vi "BINARY_DECIMAL.vi"() -> ()   [LabVIEW 2020]
panel:
  out "DECIMAL VALUE":i16
  in  "B0":bool
  in  "B1":bool
  in  "B2":bool
  in  "B3":bool
  # "BINARY TO DECIMAL"
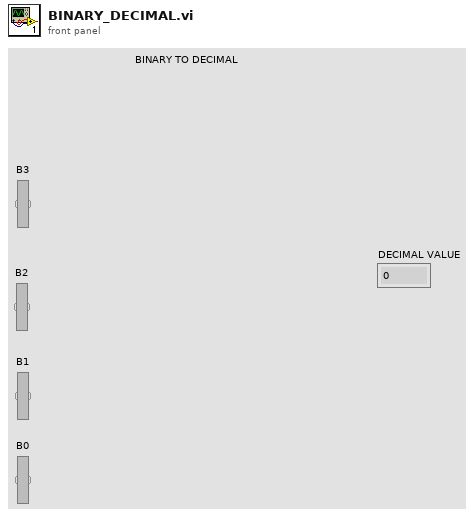
[diagram p1: front panel]
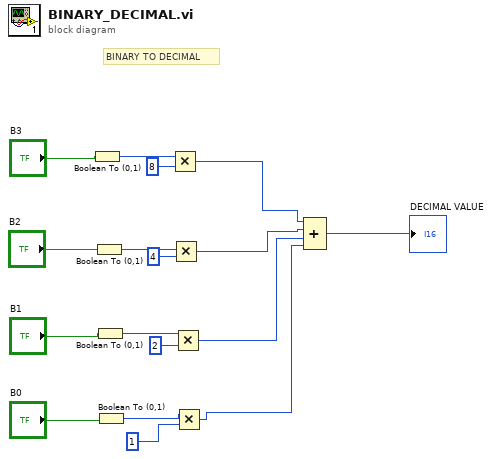
[diagram p0: block diagram]
diagram:
  # "BINARY TO DECIMAL"
  n1 = Boolean To (0,1)(Boolean="B3") -> (0, 1=w13:i16)
  n2 = Boolean To (0,1)(Boolean="B2") -> (0, 1=w9:i16)
  n3 = Boolean To (0,1)(Boolean="B1") -> (0, 1=w7:i16)
  n4 = Boolean To (0,1)(Boolean="B0") -> (0, 1=w12:i16)
  n5 = Multiply(x=w13, y=i16 8) -> (x*y=w5:i16)
  n6 = Multiply(x=w9, y=i16 4) -> (x*y=w4:i16)
  n7 = Multiply(x=w7, y=i16 2) -> (x*y=w3:i16)
  n8 = Multiply(x=w12, y=i16 1) -> (x*y=w2:i16)
  n9 = Compound Arithmetic op=ADD(w5, w4, w3, w2) -> (→"DECIMAL VALUE":i16)
